vi "Close Caller FP if In LabVIEW folder.vi"(8 "error in (no error)":errorcluster) -> (0 "error out":errorcluster)   [LabVIEW 2017]
doc: "lvAPT-User-Libraries 2022.4.27.213228\nYAO - lvAPT\nCopyright (c) 2022, lvAPT"
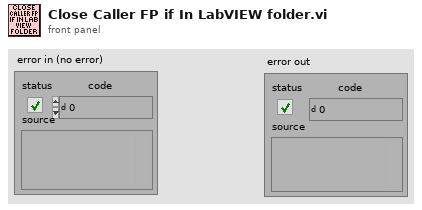
[diagram p1: front panel]
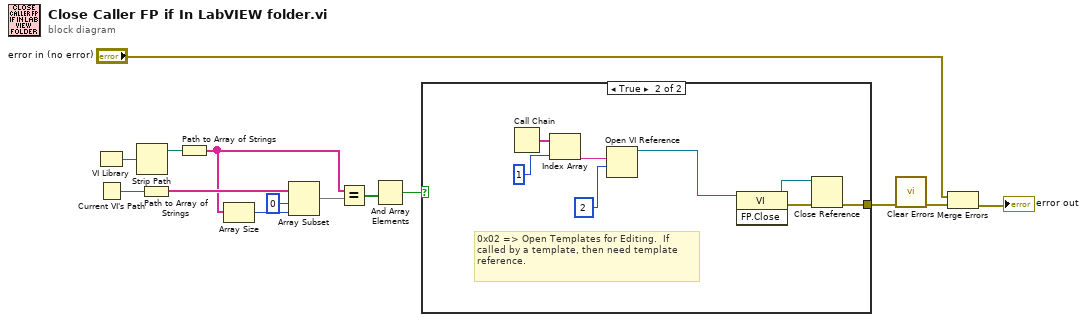
[diagram p0: block diagram]
diagram:
  n1 = VI Library() -> (path=w13:path)
  n2 = Current VI's Path() -> (path=w11:path)
  n3 = Strip Path(path=w13) -> (stripped path=w12:path)  [unwired: 1 out]
  n4 = Path to Array of Strings(0:w11) -> (2:w10:string[])  [unwired: 1 out]
  n5 = Path to Array of Strings(0:w12) -> (2:w6:string[])  [unwired: 1 out]
  n6 = Array Size(array=w6) -> (size(s)=w9:i32)
  n7 = Array Subset(array=w10, index=0, length=w9) -> (w7:string[])
  n8 = Equal?(x=w6, y=w7) -> (x = y?=w5:bool[])
  n9 = And Array Elements(Boolean array=w5) -> (logical AND=w4:bool)
  n10 = case shown="True" w4 {
    tunnel: [_ w20] -> w14
    frame False {
    }
    frame True {
      # "0x02 => Open Templates for Editing.  If called by a template, then need template reference."
      n11 = Call Chain() -> (call chain=w15:string[])
      n12 = Index Array(array=w15, index=1 ("Index")) -> (element=w17:string)
      n13 = Open VI Reference(vi path=w17, options=2) -> (vi reference=w21:refnum<vi>)  [unwired: 4 in, 1 out]
      n14 = invoke class="VI" method="FP.Close"(reference=w21) -> (reference out=w19:refnum<vi>, error out=w22:errorcluster)  [unwired: 2 in, 1 out]
      n15 = Close Reference(reference=w19, error in (no error)=w22) -> (error out=w20:errorcluster)
    }
  }
  n16 = call <vilib>:"Clear Errors.vi"("error in (no error)"=w14) -> ("error out"=w1:errorcluster)  [unwired: 5 in, 1 out]
  n17 = Merge Errors("error in (no error)", w1) -> (→"error out":errorcluster)
